vi "Teardown UE Loop.vi"(11 "Dev Actor Panel in":refnum<class "Dev Actor Panel.lvclass">) -> (0 "error out":errorcluster)   [LabVIEW 2021, in "Dev Actor Panel.lvclass"]
uses:
  Dev Actor Panel.lvclass
  Dev Actor Panel.lvclass/Dev Actor Panel.ctl
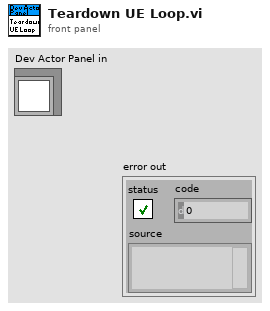
[diagram p1: front panel]
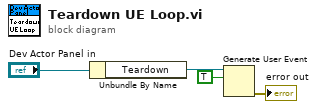
[diagram p0: block diagram]
diagram:
  n1 = Unbundle By Name("Dev Actor Panel in") -> ("Teardown"=w2:refnum<user-event>)
  n2 = Generate User Event(user event=w2, event data cluster=TRUE ("event data")) -> (error out=→"error out":errorcluster)  [unwired: 2 in, 1 out]
